vi "Create Host Stream Queues.vi"(8 "error in (no error)":errorcluster) -> (0 "error out":errorcluster, 3 "Q Refs":T1)   [LabVIEW 2019, in "CAN Stream Support Workspace Shared.lvlib"]
uses:
  CAN Stream Support Workspace Shared.lvlib
  Types/Host Stream Queue Refs.ctl
  Types/Host Stream Queue Type.ctl
  Types/Host Stream Queue Command.ctl
  <vilib>/xnet/xnet.llb/XNET Frame CAN.ctl
  <vilib>/xnet/xnet.llb/XNET Frame Type CAN.ctl
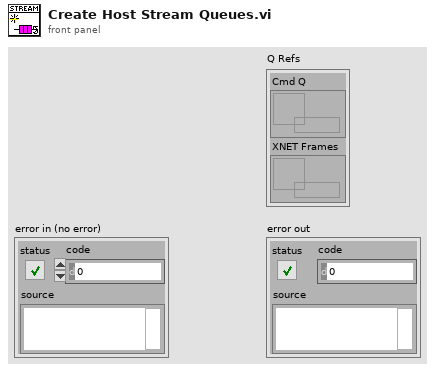
[diagram p1: front panel]
types:
  T1 = typedef "CAN Stream Support Workspace Shared.lvlib/Host Stream Queue Refs.ctl" = cluster{"Cmd Q":refnum<queue>, "XNET Frames":refnum<queue>}
  T2 = typedef "XNET Frame CAN.ctl" = cluster{"timestamp":timestamp, "payload":u8[], "identifier":u32, "type":T3, "extended?":bool, "echo?":bool}
  T3 = typedef "XNET Frame Type CAN.ctl" = u8
  T4 = typedef "CAN Stream Support Workspace Shared.lvlib/Host Stream Queue Type.ctl" = cluster{"Cmd":T5, "Target IP Address":string, "Addon":string, "Project Folder":path}
  T5 = typedef "CAN Stream Support Workspace Shared.lvlib/Host Stream Queue Command.ctl" = enum8{"Start Stream", "Stop Stream", "Exit"}
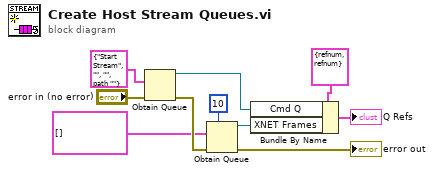
[diagram p0: block diagram]
diagram:
  n1 = Obtain Queue(element data type=T4 {"Cmd"=enum."Start Stream", "Target IP Address"="", "Addon"="", "Project Folder"=path ""}, error in (no error)="error in (no error)") -> (queue out=w2:refnum<queue>, error out=w8:errorcluster)  [unwired: 3 in, 1 out]
  n2 = Obtain Queue(max queue size (-1, unlimited)=10, element data type=T2[] [] ("Data"), error in (no error)=w8) -> (queue out=w1:refnum<queue>, error out=→"error out":errorcluster)  [unwired: 2 in, 1 out]
  n3 = Bundle By Name(cluster=T1 {"Cmd Q"=refnum, "XNET Frames"=refnum} ("Q Refs"), "Cmd Q"=w2, "XNET Frames"=w1) -> (→"Q Refs":T1)
